vi "ASIC_THx_FULL RANGO.vi"(7 "Espera acceso USB":u32, 8 "error in":errorcluster, 11 "ftHandle_in":u32) -> (0 "error out":errorcluster, 3 "ftHandle_out":u32)   [LabVIEW 2019]
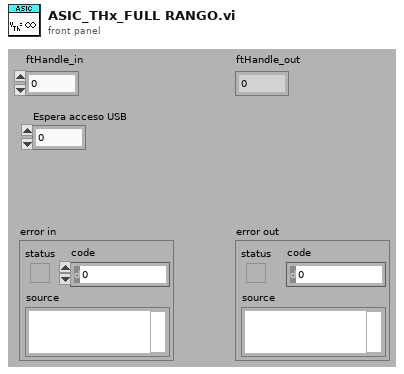
[diagram p1: front panel]
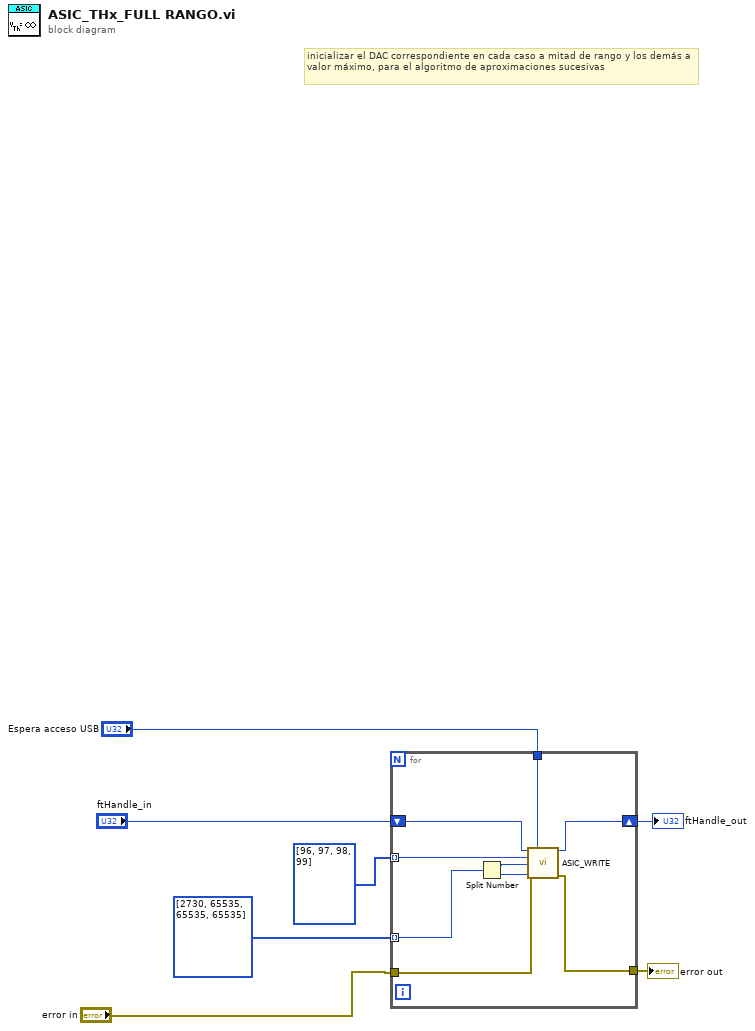
[diagram p0: block diagram]
diagram:
  # "inicializar el DAC correspondiente en cada caso a mitad de rango y los demás a valor máximo, para el algoritmo de aproximaciones sucesivas"
  n1 = for {
    shift-right: [w15] -> w2
    shift-left: "ftHandle_in" -> [w16]
    tunnel: u8[] [96, 97, 98, 99] -> [w14] mode=indexing
    tunnel: u16[] [2730, 65535, 65535, 65535] -> [w8] mode=indexing
    tunnel: "error in" -> [w13]
    tunnel: [w12] -> w5
    tunnel: "Espera acceso USB" -> [w11]
    n2 = Split Number(x=w8) -> (hi(x)=w10:u8, lo(x)=w9:u8)
    n3 = call "ASIC_WRITE.vi"("ftHandle_in"=w16, "Espera acceso USB"=w11, "Direccion Registro Asic"=w14, "Byte Alto"=w10, "Byte Bajo"=w9, "error in"=w13) -> ("ftHandle_out"=w15:u32, "error out"=w12:errorcluster)  [unwired: 8 in]
  }
  "error out" <- w5
  "ftHandle_out" <- w2
